vi "OCR-车牌识别.vi"(0 "ROI Descriptor (OCR/OCV 1)":T2={"Global Rectangle"=[455, 94, 585, 233], "Contours"=[{"ID"=enum."External", "Type"=3, "Coordinates"=[455, 94, 585, 233]}]} {"Contours"."Type" items=["No Selection", "Point", "Line", "Rectangle", "Oval", "Polygon", "Freehand Region", "Annulus", "Unused2", "Unused3", "Broken Line", "Freehand Line", "Rotated Rectangle"]}, 1 "File Path (OCR/OCV 1)":path=path "D:/Labviewprogram/视觉/视觉框架/NEW-车牌号.abc", 2 "Parameters (OCR/OCV 1)":T1={"Threshold Data"={"Method"=enum."Uniform", "Looking for"=1, "Color Mode"=0, "Kernel Size"={"Width"=32, "Height"=32}, "Ranges"=[{"Min"=1, "Max"=255}]}, "Reject Border"=TRUE, "Number Of Erosions"=0, "Size & Spacing"={"Segment Algorithm"=0, "Min Bounding Rect Width"=1, "Max Bounding Rect Width"=65536, "Min Bounding Rect Height"=1, "Max Bounding Rect Height"=65536, "Min Character Size"=20, "Max Character Size"=65536, "Min Char Spacing"=1, "Max Horiz Element Spacing"=1, "Max Vert Element Spacing"=0, "Max Space Distance"=65536}, "Read Options"={"Read Strategy"=1, "Read Resolution"=2, "Scale Dependant"=FALSE, "Aspect Ratio"=400, "Acceptance Level"=700, "Substitution Character"="?", "MultiLine"=TRUE}, "Valid Characters"=[], "Use Text Pattern"=FALSE, "Orientation"=0, "# Lines Expected"=0, "Number of Blocks"=4} {"Threshold Data"."Looking for" items=["Light on Dark", "Dark on Light"]; "Threshold Data"."Color Mode" items=["RGB", "HSL", "HSV", "HSI"]; "Size & Spacing"."Segment Algorithm" items=["None", "Shortest Segment", "Legacy Auto Split"]; "Read Options"."Read Strategy" items=["Aggressive", "Conservative"]; "Read Options"."Read Resolution" items=["Low", "Medium", "High"]; "Valid Characters"."Pre-defined characters" items=["Any Character", "User-defined Characters", "Alphabetic", "Alphanumeric", "Uppercase Letters", "Lowercase Letters", "Decimal Digits", "Hexadecimal Digits", "Pattern", "Force Space"]; "Orientation" items=["Baseline inside", "Baseline outside"]}, 7 "error in":errorcluster) -> (20 "String (OCR/OCV 1)":string, 21 "OCR Session (OCR/OCV 1)":T4, 27 "error out":errorcluster)   [LabVIEW 2018]
uses:
  <vilib>/vision/OCR.llb/IMAQ OCR Session.ctl
  <vilib>/vision/NI_Vision_Development_Module.lvlib
panel:
  out "Image Out":T3(plugin-control)
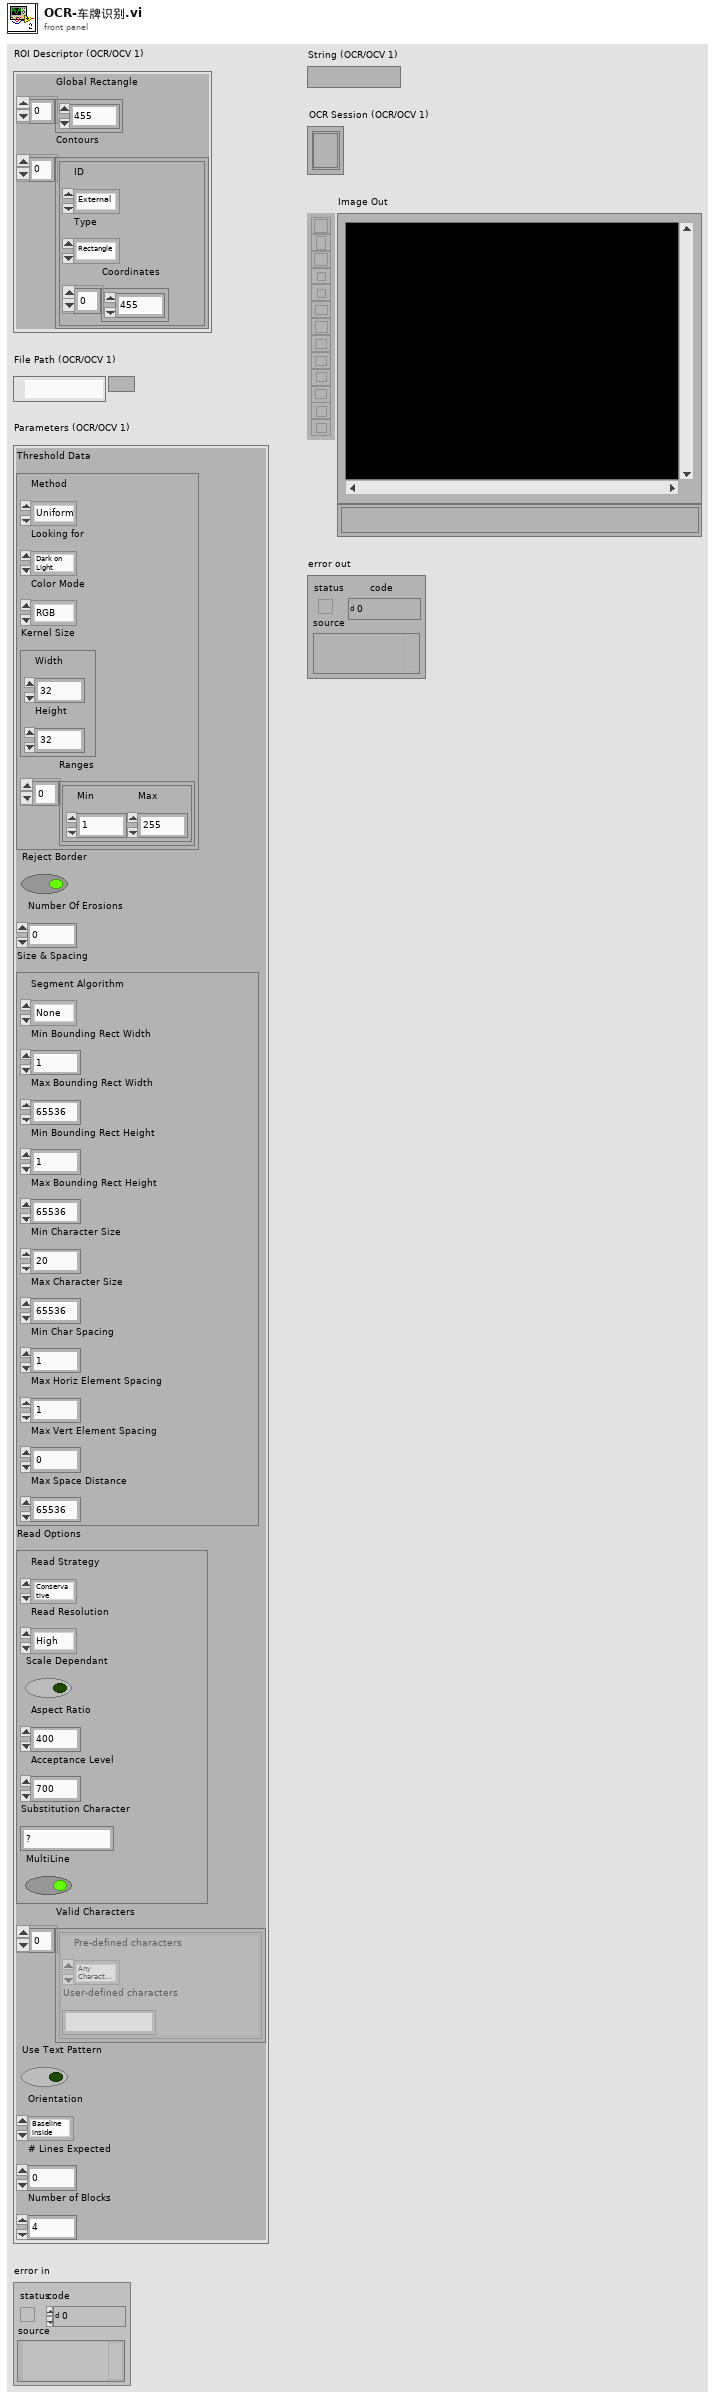
[diagram p1: front panel]
types:
  T1 = cluster{"Threshold Data":cluster{"Method":enum16{"Fixed Range", "Uniform", "Linear", "Non Linear", "Local", "Color"}, "Looking for":u32, "Color Mode":u32, "Kernel Size":cluster{"Width":i32, "Height":i32}, "Ranges":cluster{"Min":i32, "Max":i32}[]}, "Reject Border":bool, "Number Of Erosions":i32, "Size & Spacing":cluster{"Segment Algorithm":u16, "Min Bounding Rect Width":i32, "Max Bounding Rect Width":i32, "Min Bounding Rect Height":i32, "Max Bounding Rect Height":i32, "Min Character Size":i32, "Max Character Size":i32, "Min Char Spacing":i32, "Max Horiz Element Spacing":i32, "Max Vert Element Spacing":i32, "Max Space Distance":i32}, "Read Options":cluster{"Read Strategy":i32, "Read Resolution":i32, "Scale Dependant":bool, "Aspect Ratio":i32, "Acceptance Level":i32, "Substitution Character":string, "MultiLine":bool}, "Valid Characters":cluster{"Pre-defined characters":i32, "User-defined characters":string}[], "Use Text Pattern":bool, "Orientation":u32, "# Lines Expected":u32, "Number of Blocks":i32}
  T2 = cluster{"Global Rectangle":i32[], "Contours":cluster{"ID":enum32{"External", "Internal"}, "Type":u32, "Coordinates":i32[]}[]}
  T3 = typedef "IMAQ Image.ctl" = refnum<image>
  T4 = typedef "IMAQ OCR Session.ctl" = refnum<k1>
  T5 = typedef "Image Type" = u32
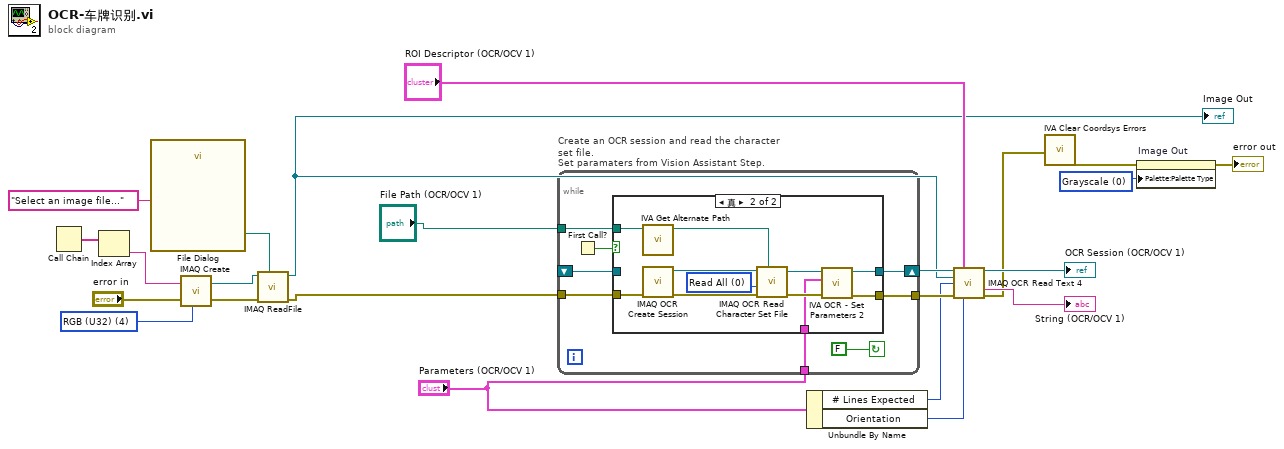
[diagram p0: block diagram]
diagram:
  w1 = u32 0 items=["Grayscale", "Binary", "Gradient", "Rainbow", "Temperature", "User Defined", "Binary 16 Bit", "Gradient 16 Bit", "Rainbow 16 Bit", "Temperature 16 Bit", "User Defined 16 Bit"] ("Palette Type")
  w15 = T5 4 items=["Grayscale (U8)", "Grayscale (I16)", "Grayscale (SGL)", "Complex (CSG)", "RGB (U32)", "HSL (U32)", "RGB (U64)", "Grayscale (U16)"] ("Image Type")
  n1 = Call Chain() -> (call chain=w19:string[])
  n2 = Index Array(array=w19) -> (element=w18:string)  [unwired: 1 in]
  n3 = call "File Dialog"("prompt"="Select an image file...") -> ("selected path"=w16:path)  [unwired: 6 in, 8 out]
  n4 = call "IMAQ Create"("Image Name"=w18, "Image Type"=w15, "error in (no error)"="error in") -> ("New Image"=w22:T3, "error out"=w21:errorcluster)  [unwired: 1 in, 1 out]
  n5 = call "IMAQ ReadFile"("File Path"=w16, "error in (no error)"=w21, "Image"=w22) -> ("error out"=w23:errorcluster, "Image Out"=w2:T3)  [unwired: 2 in, 5 out]
  "Image Out" <- w2
  n6 = while "Create an OCR session and read the character set file.\nSet paramaters from Vision Assistant Step." {
    shift-right: [w28] -> w8
    shift-left: _ -> [w27]
    tunnel: w23 -> [w30]
    tunnel: "Parameters (OCR/OCV 1)" -> [w26]
    tunnel: "File Path (OCR/OCV 1)" -> [w25]
    tunnel: [w24] -> w9
    stop <- FALSE continue-if-true
    n7 = First Call?() -> (First Call?: T/F=w29:bool)
    n8 = case "条件结构" shown="真" w29 {
      tunnel: w25 -> [_ w37]
      tunnel: w30 -> [w32 w41]
      tunnel: [w33 w39] -> w28
      tunnel: [w32 w38] -> w24
      tunnel: w26 -> [_ w34]
      tunnel: w27 -> [w33 _]
      frame False {
      }
      frame True {
        w42 = 0 items=["Read All", "Read Character Set Only", "Read Properties Only"] ("Read Options")
        n9 = call <vilib>:"IVA Get Alternate Path.vi"("Path In"=w37) -> ("Path Out"=w36:path)  [unwired: 10 out]
        n10 = call "IMAQ OCR Create Session"("error in (no error)"=w41) -> ("error out"=w43:errorcluster, "IMAQ OCR Session"=w44:T4)  [unwired: 9 out]
        n11 = call "IMAQ OCR Read Character Set File"("File Path"=w36, "error in (no error)"=w43, "Read Options"=w42, "IMAQ OCR Session"=w44) -> ("error out"=w40:errorcluster, "IMAQ OCR Session (dup)"=w35:T4)  [unwired: 1 in, 5 out]
        n12 = call <vilib>:"IVA OCR - Set Parameters 2.vi"("error in (no error)"=w40, "Parameters"=w34, "IMAQ OCR Session"=w35) -> ("error out"=w38:errorcluster, "IMAQ OCR Session Out"=w39:T4)  [unwired: 7 in]
      }
    }
  }
  n13 = Unbundle By Name("Parameters (OCR/OCV 1)") -> ("# Lines Expected"=w6:u32, "Orientation"=w7:u32)
  n14 = call "IMAQ OCR Read Text 4"("IMAQ OCR Session"=w8, "ROI Descriptor"="ROI Descriptor (OCR/OCV 1)", "Image"=w2, "Number of Lines Requested"=w6, "error in (no error)"=w9, "Orientation"=w7) -> ("IMAQ OCR Session (dup)"=→"OCR Session (OCR/OCV 1)":T4, "Read String"=→"String (OCR/OCV 1)":string, "error out"=w5:errorcluster)  [unwired: 7 out]
  n15 = call <vilib>:"IVA Clear Coordsys Errors.vi"("error in (no error)"=w5) -> ("error out"=w4:errorcluster)  [unwired: 10 in]
  n16 = property on="Image Out" class="ImageControl"(error in=w4, "Palette:Palette Type"=w1) -> (error out=→"error out":errorcluster)  [unwired: 1 in, 1 out]
